vi "Save Freq List.vi"(6 "Spec List":cluster{"Lower":dbl, "Upper":dbl}[](array[cluster]), 8 "error in (no error)":errorcluster, 10 "correctedFreqList":T1(array[cluster]), 11 "Freq List file":path) -> (0 "error out":errorcluster)   [LabVIEW 2018]
uses:
  <vilib>/Utility/file.llb/Write Delimited Spreadsheet (DBL).vi
panel:
  out "appended array":dbl[][](array[numeric])
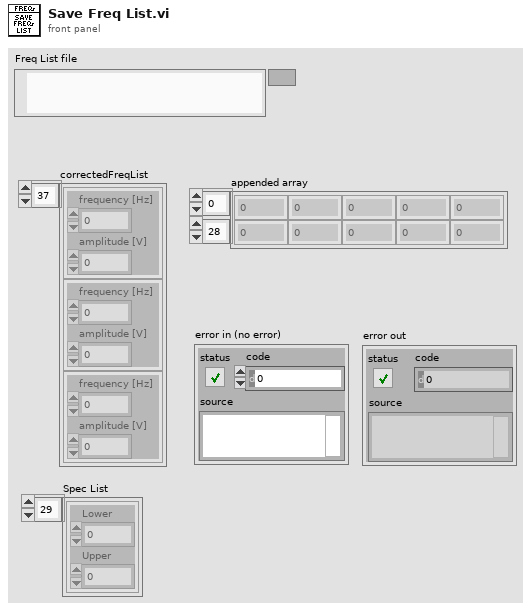
[diagram p1: front panel]
types:
  T1 = cluster{"frequency [Hz]":dbl, "amplitude [V]":dbl}[]
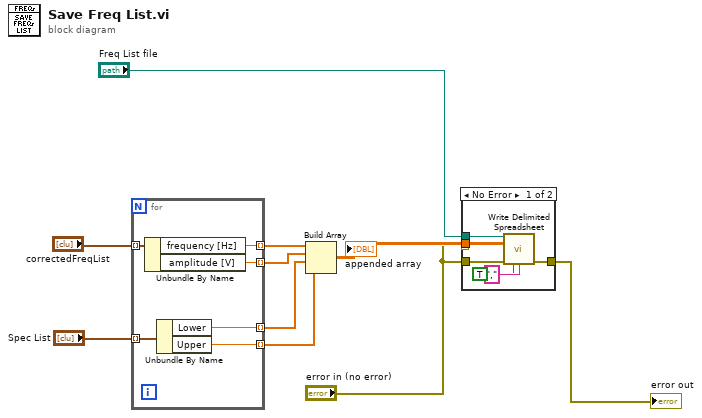
[diagram p0: block diagram]
diagram:
  n1 = for {
    tunnel: "correctedFreqList" -> [w16] mode=indexing
    tunnel: [w15] -> w9 mode=indexing
    tunnel: [w14] -> w8 mode=indexing
    tunnel: "Spec List" -> [w13] mode=indexing
    tunnel: [w12] -> w2 mode=indexing
    tunnel: [w11] -> w1 mode=indexing
    n2 = Unbundle By Name(w16) -> ("frequency [Hz]"=w15:dbl, "amplitude [V]"=w14:dbl)
    n3 = Unbundle By Name(w13) -> ("Lower"=w12:dbl, "Upper"=w11:dbl)
  }
  n4 = Build Array(w9, w8, w2, w1) -> (w6:dbl[][])
  "appended array" <- w6
  n5 = case shown="No Error" "error in (no error)" {
    tunnel: "Freq List file" -> [w22 _]
    tunnel: w6 -> [w21 _]
    tunnel: "error in (no error)" -> [w20 w23]
    tunnel: [w19 w23] -> w5
    frame No Error {
      n6 = call-poly <vilib>:"Write Delimited Spreadsheet.vi"("file path (dialog if empty)"=w22, "2D data"=w21, "error in (no error)"=w20, "transpose? (no:F)"=TRUE, "delimiter (\\t)"="," ("delimiter (\\t)")) -> ("error out"=w19:errorcluster)  [unwired: 9 in, 1 out]
    }
    frame Error {
    }
  }
  "error out" <- w5
